vi "TAT_Start.vi"(8 "error In":errorcluster) -> (0 "error out":errorcluster)   [LabVIEW 2017]
uses:
  Controls/Ass. Loop Control.ctl
  <vilib>/addons/database/NI_Database_API.lvlib
  <vilib>/Utility/error.llb/DialogType.ctl
  <vilib>/addons/database/Connection.llb/DB Tools Open Connec (Path).vi
panel:
  out "USER:-":string
  in  "Stop":bool
  out "DATE/TIME":string
  # "Nm"
  # "UNIQUE CIRCLE\nAUTOMATION Pvt Ltd"
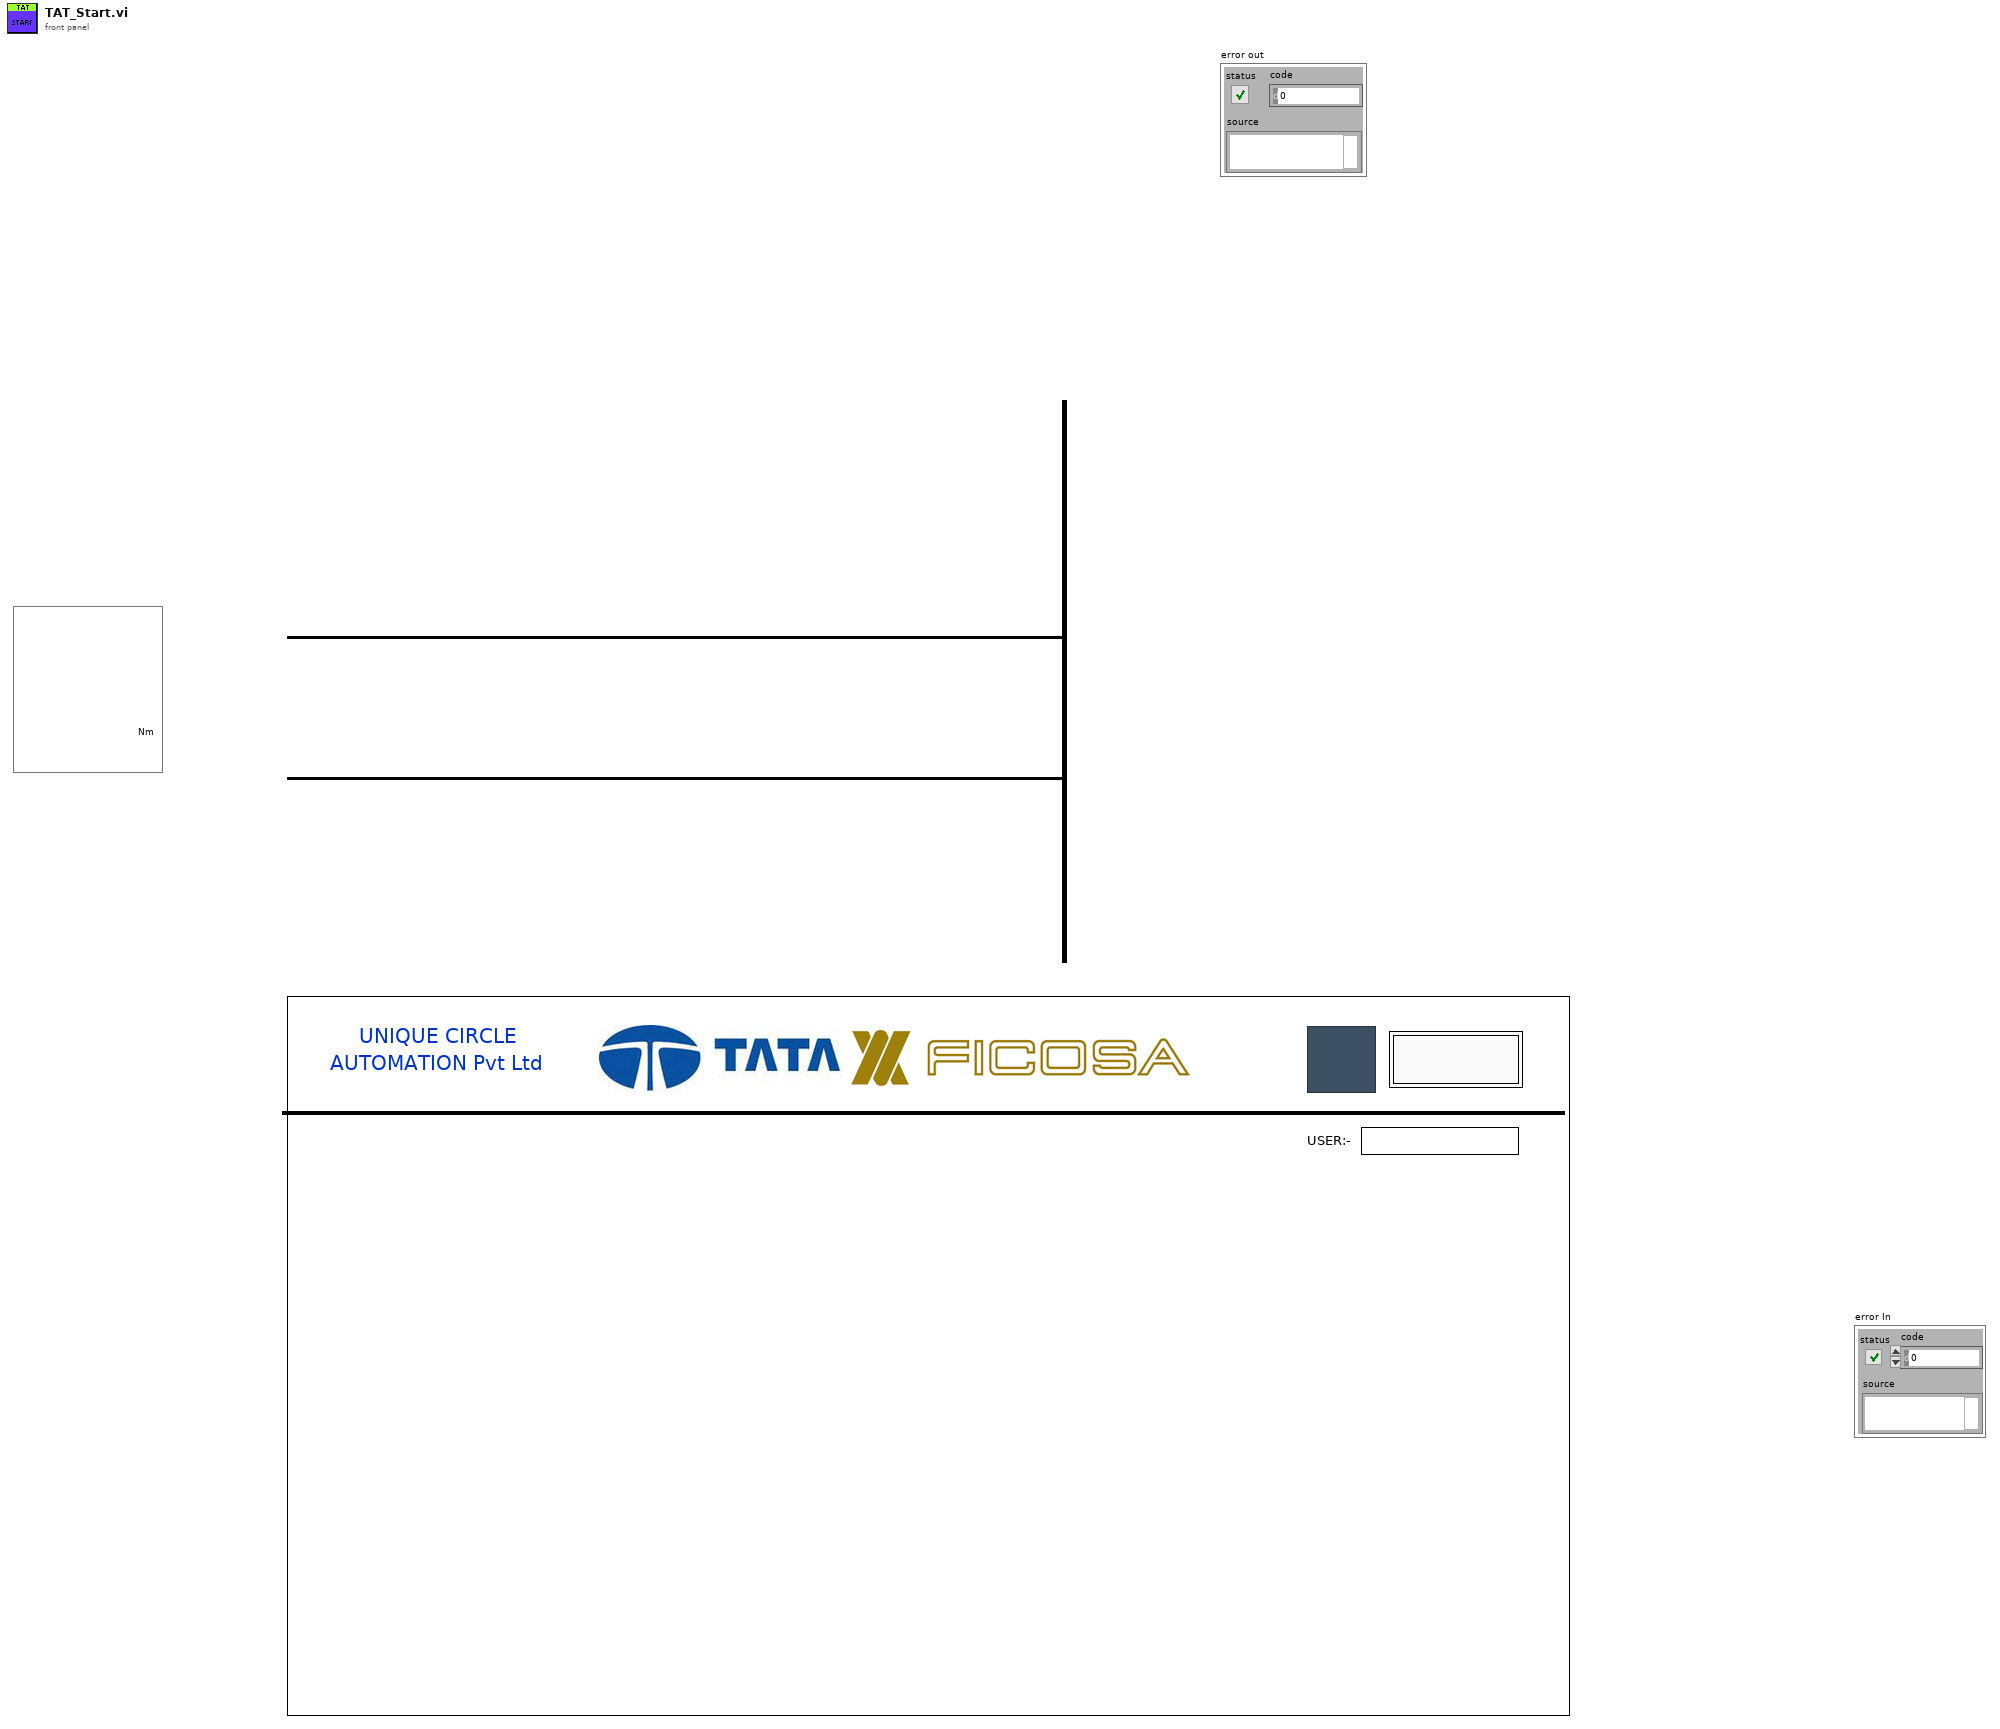
[diagram p1: front panel]
types:
  T1 = typedef "DialogType.ctl" = u16
  T2 = typedef "Ass. Loop Control.ctl" = enum16{"Package_Qty_Count", "GENERATE_QR_PRNT", "Cluster_update", "Waiting_for_scan", "barcode CHECK", "Int", "SaveReport ", "Barcode Print", "Start Cycle", "Wait", "Cycle End", "Stop"}
  T3 = enum32{"invalid app kind", "Development System", "Run Time System", "Student Edition", "Embedded LabVIEW", "Evaluation", "Custom"}
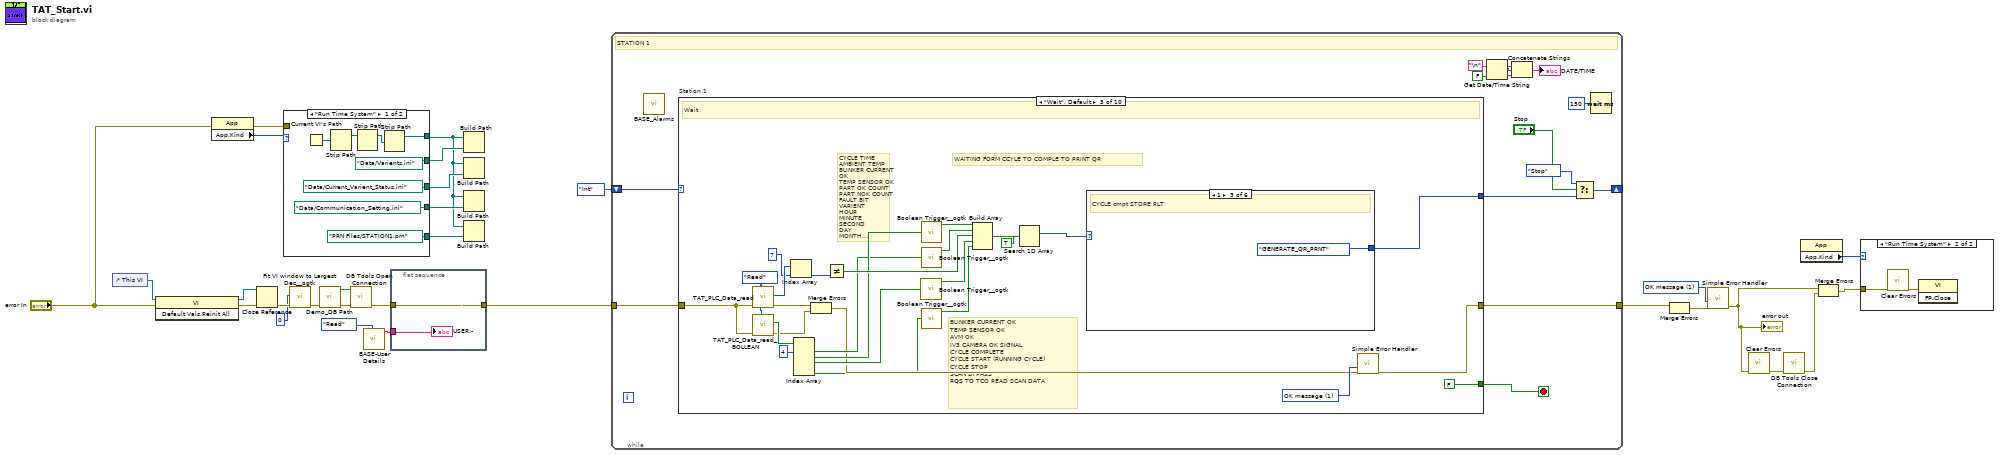
[diagram p0: block diagram]
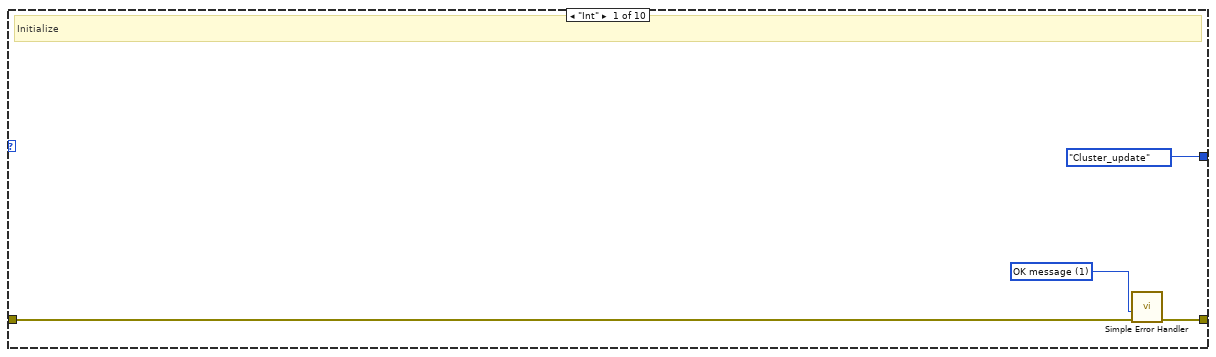
[diagram p3: hidden frame]
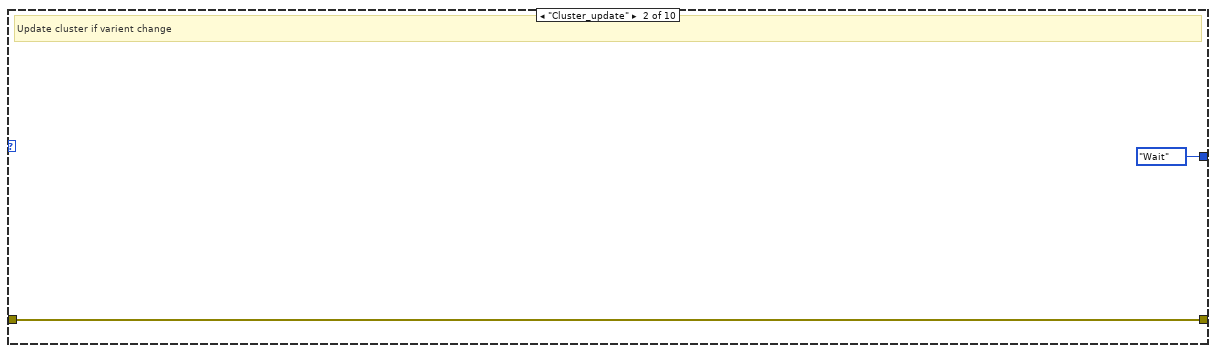
[diagram p4: hidden frame]
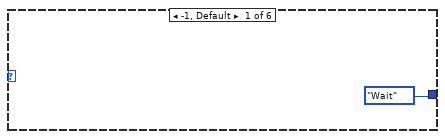
[diagram p5: hidden frame]
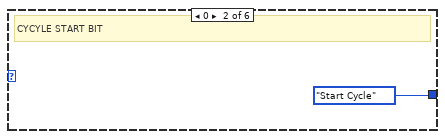
[diagram p6: hidden frame]
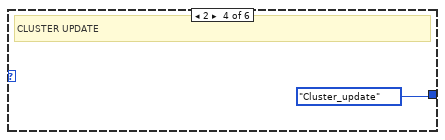
[diagram p7: hidden frame]
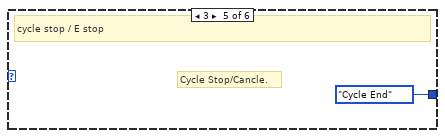
[diagram p8: hidden frame]
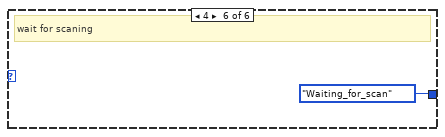
[diagram p9: hidden frame]
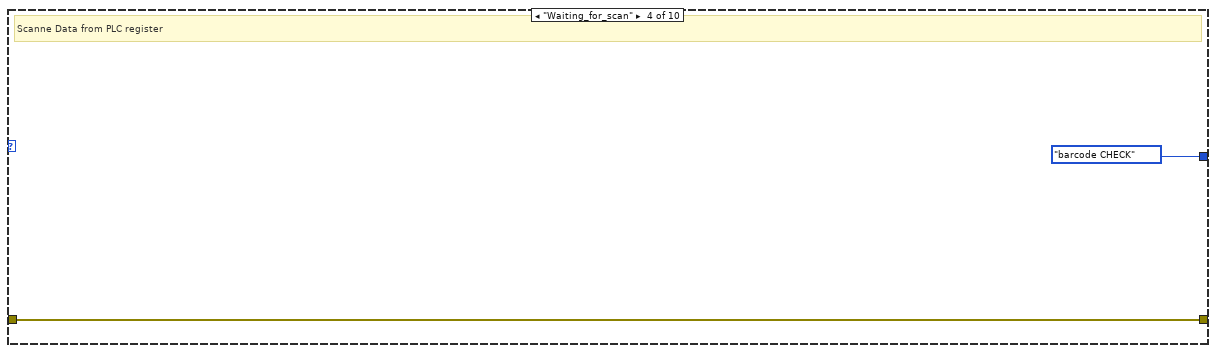
[diagram p10: hidden frame]
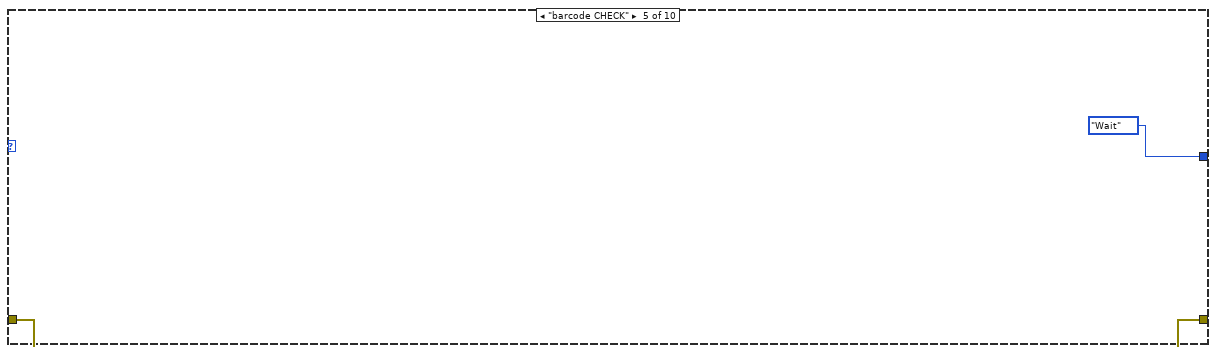
[diagram p11: hidden frame]
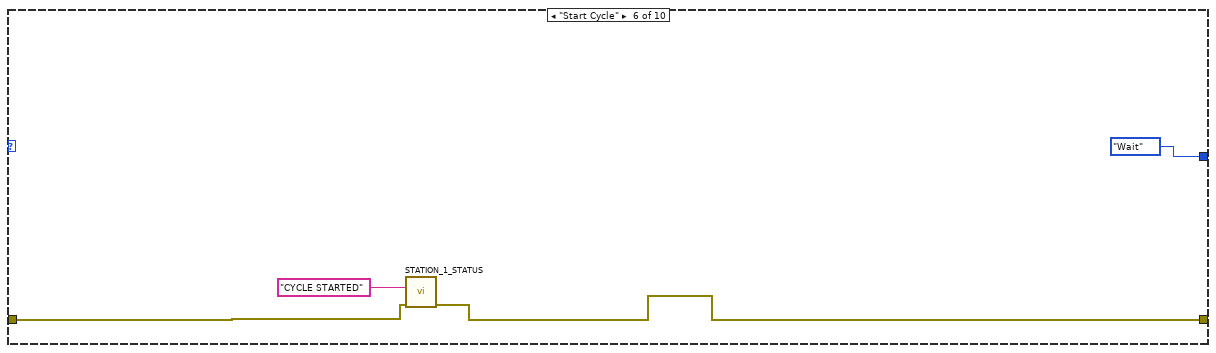
[diagram p12: hidden frame]
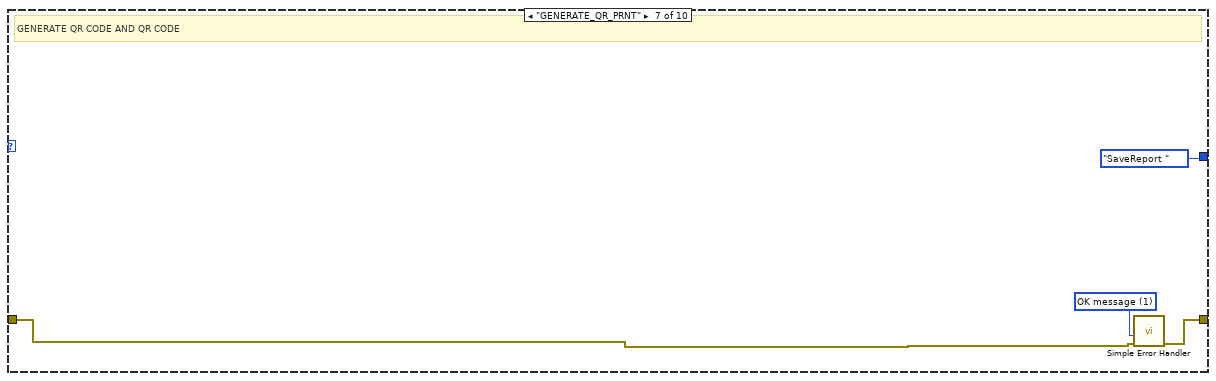
[diagram p13: hidden frame]
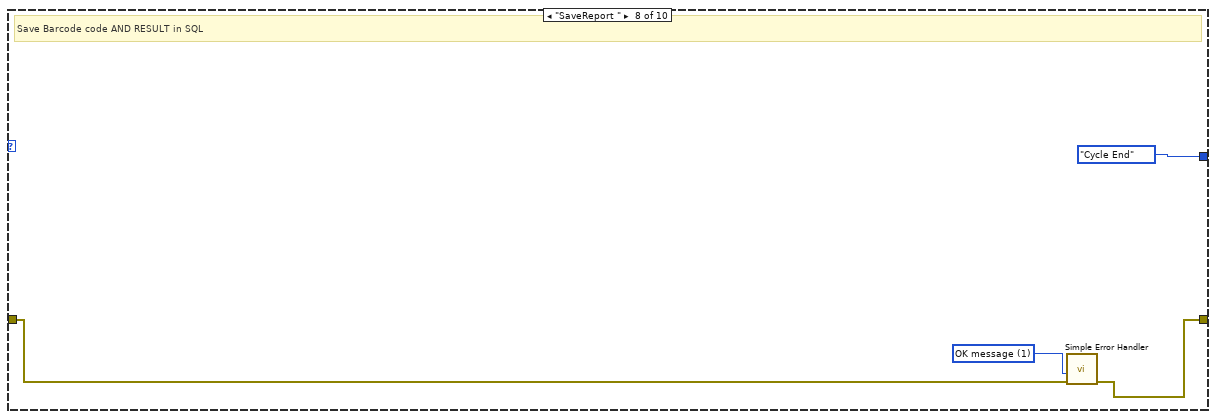
[diagram p14: hidden frame]
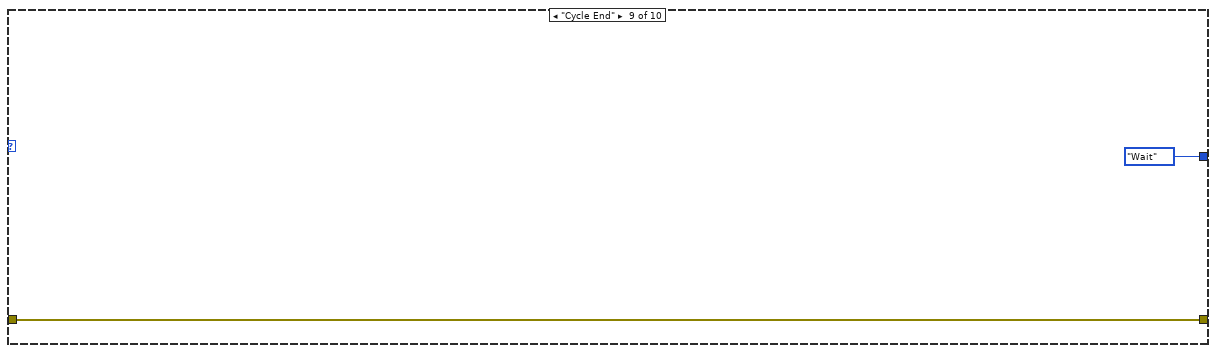
[diagram p15: hidden frame]
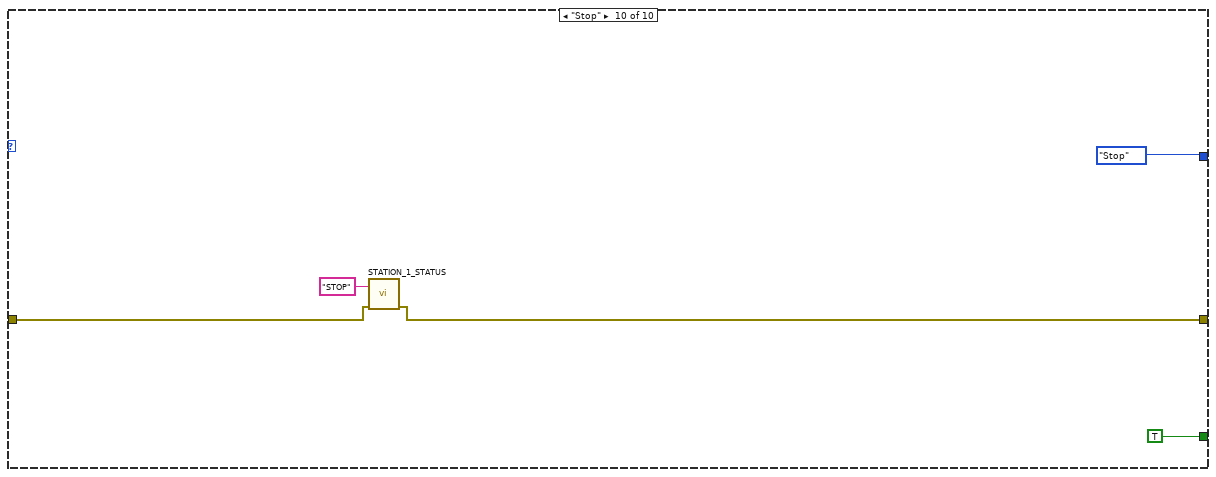
[diagram p16: hidden frame]
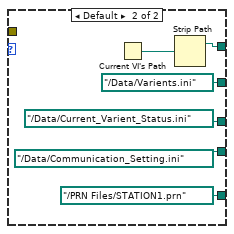
[diagram p17: hidden frame]
diagram:
  w20 = T1 1 items=["no dialog", "OK message", "continue or stop message", "OK message + warnings", "continue/stop + warnings"] ("type of dialog (OK msg:1)")
  n1 = control-ref of="This VI"() -> (w29:refnum<vi>)
  n2 = invoke class="VI" method="Default Vals.Reinit All"(reference=w29, error in="error In") -> (reference out=w27:refnum<vi>, error out=w28:errorcluster)  [unwired: 1 in, 1 out]
  n3 = property class="App"(error in="error In") -> (error out=w14:errorcluster, "App.Kind"=w18:T3)  [unwired: 1 in, 1 out]
  n4 = Close Reference(reference=w27, error in (no error)=w28) -> (error out=w26:errorcluster)
  n5 = case shown="\"Run Time System\"" w18 {
    tunnel: [path "Data/Varients.ini" ("path") path "../Data/Varients.ini" ("path")] -> w17
    tunnel: [w33 w41] -> w3
    tunnel: [path "Data/Current_Varient_Status.ini" ("path") path "../Data/Current_Varient_Status.ini" ("path")] -> w16
    tunnel: [path "Data/Communication_Setting.ini" ("path") path "../Data/Communication_Setting.ini" ("path")] -> w15
    tunnel: w14 -> [_ _]
    tunnel: [path "PRN Files/STATION1.prn" ("path") path "../PRN Files/STATION1.prn" ("path")] -> w12
    frame "Run Time System" {
      n6 = Current VI's Path() -> (path=w36:path)
      n7 = Strip Path(path=w36) -> (stripped path=w35:path)  [unwired: 1 out]
      n8 = Strip Path(path=w35) -> (stripped path=w34:path)  [unwired: 1 out]
      n9 = Strip Path(path=w34) -> (stripped path=w33:path)  [unwired: 1 out]
    }
    frame Default {
      n10 = Current VI's Path() -> (path=w42:path)
      n11 = Strip Path(path=w42) -> (stripped path=w41:path)  [unwired: 1 out]
    }
  }
  n12 = call <userlib>:"Fit VI window to Largest Dec__ogtk.vi"("error in (no error)"=w26, "border spacing (2 px)"=0) -> ("error out"=w9:errorcluster)  [unwired: 4 in, 1 out]
  n13 = call "Demo_DB Path.vi"("error in"=w9) -> ("error out"=w11:errorcluster, "DB Path"=w10:path)  [unwired: 9 in]
  n14 = call-poly <vilib>:"DB Tools Open Connection.vi"("error in (no error)"=w11, "connection information"=w10) -> ("error out"=w8:errorcluster)  [unwired: 6 in, 1 out]
  n15 = call "BASE-User Details.vi"("Enum"=enum16{"Read", "Write"}."Read") -> ("User Name Out"=w21:string)  [unwired: 9 in, 1 out]
  n16 = flat-sequence {
    tunnel: [w45] -> w2
    tunnel: w8 -> [w45]
    tunnel: w21 -> [w44]
    frame #0 {
      "USER:-" <- w44
    }
  }
  n17 = Build Path(base path=w3, name or relative path=w17) -> ()  [unwired: 1 out]
  n18 = Build Path(base path=w3, name or relative path=w16) -> ()  [unwired: 1 out]
  n19 = Build Path(base path=w3, name or relative path=w15) -> ()  [unwired: 1 out]
  n20 = Build Path(base path=w3, name or relative path=w12) -> ()  [unwired: 1 out]
  n21 = while {
    tunnel: w2 -> [w46]
    shift-right: [w56] -> _
    shift-left: Ass._Loop_Control."Int" ("Enum") -> [w59]
    tunnel: [w57] -> w24
    stop <- w49 stop-if-true
    # "STATION 1"
    n22 = call "BASE_Alarms.vi"() -> ()  [unwired: 11 in, 1 out]
    n23 = case "Station 1" shown="\"Wait\", Default" w59 {
      tunnel: [Ass._Loop_Control."Cluster_update" ("Enum") Ass._Loop_Control."Wait" ("Enum") w84 Ass._Loop_Control."barcode CHECK" ("Enum") Ass._Loop_Control."Wait" ("Enum") Ass._Loop_Control."Wait" ("Enum") Ass._Loop_Control."SaveReport " ("Enum") Ass._Loop_Control."Cycle End" ("Enum") Ass._Loop_Control."Wait" ("Enum") Ass._Loop_Control."Stop" ("Enum")] -> w48
      tunnel: [_ _ FALSE _ _ _ _ _ _ TRUE] -> w49
      tunnel: [w61 w64 w81 w98 w100 w102 w108 w111 w114 w116] -> w57
      tunnel: w46 -> [w60 w64 w78 w98 w100 w103 w106 w110 w114 w117]
      frame "Int" {
        w62 = T1 1 items=["no dialog", "OK message", "continue or stop message", "OK message + warnings", "continue/stop + warnings"] ("type of dialog (OK msg:1)")
        # "Initialize"
        n24 = call <vilib>:"Simple Error Handler.vi"("type of dialog (OK msg:1)"=w62, "error in (no error)"=w60) -> ("error out"=w61:errorcluster)  [unwired: 3 in, 4 out]
      }
      frame "Cluster_update" {
        # "Update cluster if varient change"
      }
      frame "Wait", Default {
        w82 = T1 1 items=["no dialog", "OK message", "continue or stop message", "OK message + warnings", "continue/stop + warnings"] ("type of dialog (OK msg:1)")
        w79 = enum16{"Read", "Write"}."Read" ("Enum")
        # "CYCLE TIME\nAMBIENT TEMP\nBLINKER CURRENT OK\nTEMP SENSOR OK\nPART OK COUNT\nPART NOK COUNT\nFAULT BIT\nVARIENT\nHOUR\nMINUTE\nSECOND\nDAY\nMONTH\nYEAR\nSERIAL NUMBER"
        # "BLINKER CURRENT OK\nTEMP SENSOR OK\nAVM OK\nIV3 CAMERA OK SIGNAL\nCYCLE COMPLETE\nCYCLE START (RUNNING CYCLE)\nCYCLE STOP\nSCAN BYPASS\nRQS TO TCO READ SCAN DATA"
        # "WAITING FORM CCYLE TO COMPLE TO PRINT QR"
        # "Wait"
        n25 = call "TAT_PLC_Data_read.vi"("Enum"=w79, "error in (no error)"=w78) -> ("error out"=w69:errorcluster, "Array 2"=w85:u16[])  [unwired: 8 in]
        n26 = call "TAT_PLC_Data_read_BOLLEAN.vi"("Enum"=w79, "error in (no error)"=w78) -> ("error out"=w67:errorcluster, "Array 2"=w77:bool[])  [unwired: 8 in]
        n27 = Index Array(array=w85, index=7) -> (element=w86:u16)
        n28 = Index Array(array=w77, index #1=4 ("index")) -> (element #1=w74:bool, element #2=w75:bool, element #3=w73:bool, element #5=w66:bool)  [unwired: 4 in, 1 out]
        n29 = Merge Errors(w69, w67) -> (w68:errorcluster)
        n30 = Not Equal?(y=w86) -> (x != y?=w83:bool)  [unwired: 1 in]
        n31 = call <userlib>:"Boolean Trigger__ogtk.vi"("Boolean Input"=w73) -> ("Rising Edge"=w72:bool)  [unwired: 1 in, 1 out]
        n32 = call <userlib>:"Boolean Trigger__ogtk.vi"("Boolean Input"=w75) -> ("Rising Edge"=w90:bool)  [unwired: 1 in, 1 out]
        n33 = call <userlib>:"Boolean Trigger__ogtk.vi"("Boolean Input"=w74) -> ("Rising Edge"=w80:bool)  [unwired: 1 in, 1 out]
        n34 = call <userlib>:"Boolean Trigger__ogtk.vi"("Boolean Input"=w66) -> ("Rising Edge"=w71:bool)  [unwired: 1 in, 1 out]
        n35 = Build Array(w90, w80, w83, w72, w71) -> (w89:bool[])
        n36 = Search 1D Array(1D array=w89, element=TRUE ("Boolean Input")) -> (index of element=w88:i32)  [unwired: 1 in]
        n37 = case shown="1" w88 {
          tunnel: [Ass._Loop_Control."Wait" ("Enum") Ass._Loop_Control."Start Cycle" ("Enum") Ass._Loop_Control."GENERATE_QR_PRNT" ("Enum") Ass._Loop_Control."Cluster_update" ("Enum") Ass._Loop_Control."Cycle End" ("Enum") Ass._Loop_Control."Waiting_for_scan" ("Enum")] -> w84
          frame -1, Default {
          }
          frame 0 {
            # "CYCYLE START BIT"
          }
          frame 1 {
            # "CYCLE cmpt STORE RLT"
          }
          frame 2 {
            # "CLUSTER UPDATE"
          }
          frame 3 {
            # "Cycle Stop/Cancle."
            # "cycle stop / E stop"
          }
          frame 4 {
            # "wait for scaning"
          }
        }
        n38 = call <vilib>:"Simple Error Handler.vi"("type of dialog (OK msg:1)"=w82, "error in (no error)"=w68) -> ("error out"=w81:errorcluster)  [unwired: 3 in, 4 out]
      }
      frame "Waiting_for_scan" {
        # "Scanne Data from PLC register"
      }
      frame "barcode CHECK" {
      }
      frame "Start Cycle" {
        n39 = call "STATION_1_STATUS.vi"("error in (no error)"=w103, "STATUS"="CYCLE STARTED" ("Cycle Status")) -> ("error out"=w102:errorcluster)  [unwired: 9 in]
      }
      frame "GENERATE_QR_PRNT" {
        w109 = T1 1 items=["no dialog", "OK message", "continue or stop message", "OK message + warnings", "continue/stop + warnings"] ("type of dialog (OK msg:1)")
        # "GENERATE QR CODE AND QR CODE"
        n40 = call <vilib>:"Simple Error Handler.vi"("type of dialog (OK msg:1)"=w109, "error in (no error)"=w106) -> ("error out"=w108:errorcluster)  [unwired: 3 in, 4 out]
      }
      frame "SaveReport " {
        w112 = T1 1 items=["no dialog", "OK message", "continue or stop message", "OK message + warnings", "continue/stop + warnings"] ("type of dialog (OK msg:1)")
        # "Save Barcode code AND RESULT in SQL"
        n41 = call <vilib>:"Simple Error Handler.vi"("type of dialog (OK msg:1)"=w112, "error in (no error)"=w110) -> ("error out"=w111:errorcluster)  [unwired: 3 in, 4 out]
      }
      frame "Cycle End" {
      }
      frame "Stop" {
        n42 = call "STATION_1_STATUS.vi"("error in (no error)"=w117, "STATUS"="STOP" ("Cycle Status")) -> ("error out"=w116:errorcluster)  [unwired: 9 in]
      }
    }
    n43 = Get Date/Time String(want seconds? (F)=FALSE) -> (date string=w53:string, time string=w52:string)  [unwired: 2 in]
    n44 = Concatenate Strings(w53, "\n", w52) -> (→"DATE/TIME":string)
    n45 = Select(t=Ass._Loop_Control."Stop" ("Enum"), s="Stop", f=w48) -> (s? t:f=w56:T2)
    n46 = Wait (ms)(milliseconds to wait=u32 150) -> ()  [unwired: 1 out]
  }
  n47 = Merge Errors(w24) -> (w23:errorcluster)  [unwired: 1 in]
  n48 = call <vilib>:"Simple Error Handler.vi"("type of dialog (OK msg:1)"=w20, "error in (no error)"=w23) -> ("error out"=w4:errorcluster)  [unwired: 3 in, 4 out]
  "error out" <- w4
  n49 = call <vilib>:"Clear Errors.vi"("error in (no error)"=w4) -> ("error out"=w1:errorcluster)  [unwired: 5 in, 1 out]
  n50 = call <vilib>:"DB Tools Close Connection.vi"("error in (no error)"=w1) -> ("error out"=w5:errorcluster)  [unwired: 6 in]
  n51 = property class="App"() -> ("App.Kind"=w19:T3)  [unwired: 2 in, 2 out]
  n52 = Merge Errors(w4, w5) -> (w6:errorcluster)
  n53 = case shown="\"Run Time System\"" w19 {
    tunnel: w6 -> [_ w122]
    frame "invalid app kind", Default {
    }
    frame "Run Time System" {
      n54 = call <vilib>:"Clear Errors.vi"("error in (no error)"=w122) -> ("error out"=w121:errorcluster)  [unwired: 5 in, 1 out]
      n55 = invoke class="VI" method="FP.Close"(error in=w121) -> ()  [unwired: 2 in, 3 out]
    }
  }
